vi "Bernoulli CDF.vi"(9 "p":dbl=0.2, 11 "x":dbl) -> (0 "error":i32, 3 "cdf(x)":dbl=0.8)   [LabVIEW 2017, in "NI_Gmath.lvlib"]
doc: "Computes the discrete cumulative distribution function (CDF), or the probability that the random variate X, where X describes the selected distribution type, takes on a value less than or equal to <B>x</B>. You must manually select the polymorphic instance to use."
uses:
  NI_Gmath.lvlib
  st_error_code.ctl
panel:
  # "Bernoulli CDF"
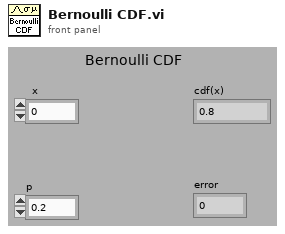
[diagram p1: front panel]
types:
  T1 = typedef "NI_Gmath.lvlib/st_error_code.ctl" = i32
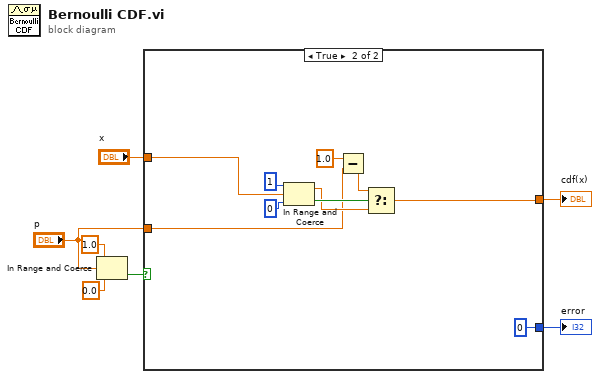
[diagram p0: block diagram]
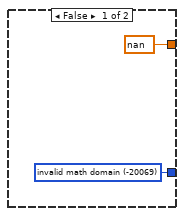
[diagram p2: hidden frame]
diagram:
  n1 = In Range and Coerce(upper limit=1.0, x="p", lower limit=0.0) -> (In Range?=w5:bool)  [unwired: 1 out]
  n2 = case shown="True" w5 {
    tunnel: [w8 0 ("invalid math domain")] -> w2
    tunnel: "p" -> [_ w10]
    tunnel: "x" -> [_ w16]
    tunnel: [nan w11] -> w1
    frame False {
      w8 = T1 -20069 items=["invalid math domain"=-20069, "Fourier interpolation size m >= n"=-20070, "empty array"=-20003] ("stat interp error code")
    }
    frame True {
      n3 = In Range and Coerce(upper limit=1, x=w16, lower limit=0) -> (coerced(x)=w12:dbl, In Range?=w14:bool)
      n4 = Subtract(x=1.0, y=w10) -> (x-y=w13:dbl)
      n5 = Select(t=w13, s=w14, f=w12) -> (s? t:f=w11:dbl)
    }
  }
  "cdf(x)" <- w1
  "error" <- w2
